vi "indexed_cache_analog.vi"(2 "new_val":fxp<+/-,24,5>, 5 "index":fxp<+,3,3>) -> (20 "$val_0":fxp<+/-,24,5>, 21 "$val_1":fxp<+/-,24,5>, 22 "$val_2":fxp<+/-,24,5>, 23 "$val_3":fxp<+/-,24,5>, 24 "$val_4":fxp<+/-,24,5>, 25 "$val_5":fxp<+/-,24,5>, 26 "$val_6":fxp<+/-,24,5>, 27 "$val_7":fxp<+/-,24,5>)   [LabVIEW 2018]
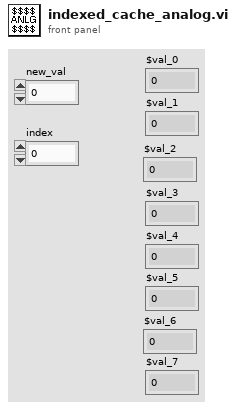
[diagram p1: front panel]
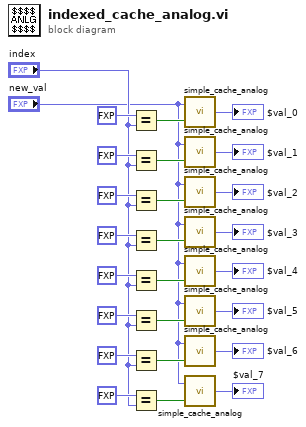
[diagram p0: block diagram]
diagram:
  n1 = Equal?(x=fxp<+,1,1> 0.0, y="index") -> (x = y?=w17:bool)
  n2 = Equal?(x=fxp<+,1,1> 1.0, y="index") -> (x = y?=w16:bool)
  n3 = Equal?(x=fxp<+,1,2> 2.0, y="index") -> (x = y?=w15:bool)
  n4 = Equal?(x=fxp<+,2,2> 3.0, y="index") -> (x = y?=w14:bool)
  n5 = Equal?(x=fxp<+,1,3> 4.0, y="index") -> (x = y?=w13:bool)
  n6 = Equal?(x=fxp<+,3,3> 5.0, y="index") -> (x = y?=w12:bool)
  n7 = Equal?(x=fxp<+,2,3> 6.0, y="index") -> (x = y?=w11:bool)
  n8 = Equal?(x=fxp<+,3,3> 7.0, y="index") -> (x = y?=w10:bool)
  n9 = call "simple_cache_analog.vi"("refresh"=w17, "new_val"="new_val") -> ("$_val"=→"$val_0":fxp<+/-,24,5>)
  n10 = call "simple_cache_analog.vi"("refresh"=w16, "new_val"="new_val") -> ("$_val"=→"$val_1":fxp<+/-,24,5>)
  n11 = call "simple_cache_analog.vi"("refresh"=w15, "new_val"="new_val") -> ("$_val"=→"$val_2":fxp<+/-,24,5>)
  n12 = call "simple_cache_analog.vi"("refresh"=w14, "new_val"="new_val") -> ("$_val"=→"$val_3":fxp<+/-,24,5>)
  n13 = call "simple_cache_analog.vi"("refresh"=w13, "new_val"="new_val") -> ("$_val"=→"$val_4":fxp<+/-,24,5>)
  n14 = call "simple_cache_analog.vi"("refresh"=w12, "new_val"="new_val") -> ("$_val"=→"$val_5":fxp<+/-,24,5>)
  n15 = call "simple_cache_analog.vi"("refresh"=w11, "new_val"="new_val") -> ("$_val"=→"$val_6":fxp<+/-,24,5>)
  n16 = call "simple_cache_analog.vi"("refresh"=w10, "new_val"="new_val") -> ("$_val"=→"$val_7":fxp<+/-,24,5>)
